vi "Main.vi"   [LabVIEW 2019]
uses:
  SampleCommonLib.lvlib
  SampleClass/SampleClass.lvclass
  ExternalClass/ExternalClass.lvclass
  ExternalDep/ExternalDepClass/ExternalDepClass.lvclass
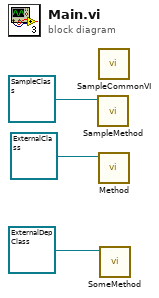
[diagram p0: block diagram]
diagram:
  n1 = call-dynamic "SampleMethod.vi"("SampleClass in"=refnum<class "SampleClass.lvclass"> refnum) -> ()  [unwired: 9 in, 2 out]
  n2 = call "SampleCommonVI.vi"() -> ()  [unwired: 12 in]
  n3 = call-dynamic "Method.vi"("ExternalClass in"=refnum<class "ExternalClass.lvclass"> refnum) -> ()  [unwired: 9 in, 2 out]
  n4 = call-dynamic "SomeMethod.vi"("ExternalDepClass in"=refnum<class "ExternalDepClass.lvclass"> refnum ("ExternalDep.lvlib:ExternalDepClass.lvclass")) -> ()  [unwired: 9 in, 2 out]
